vi "AddControlArray.vi"(8 "error in (no error)":errorcluster, 9 "CtlRef Array":refnum<vi>[](array[refnum]), 10 "CtlLabel Array":string[](array[string]), 11 "CtlLookup In":T1) -> (0 "error out":errorcluster, 3 "CtlLookup Out":T1)   [LabVIEW 2020, in "CtlReferences.lvlib" / "CtlReferences.lvclass"]
uses:
  CtlReferences.lvclass
  TypeDefs/CtlLookup.ctl
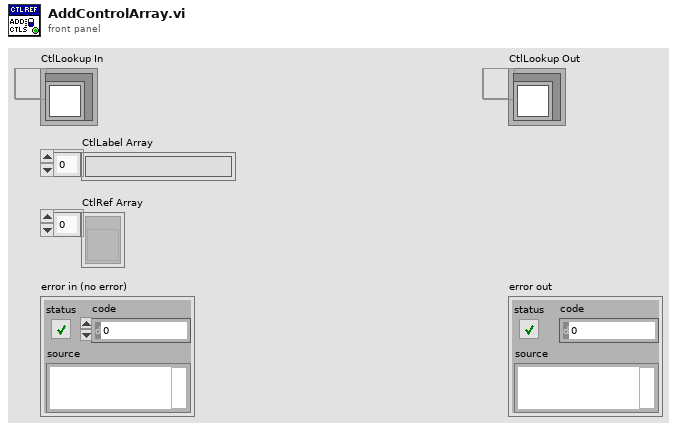
[diagram p1: front panel]
types:
  T1 = typedef "CtlReferences.lvlib/CtlReferences.lvclass/CtlLookup.ctl" = refnum<data-value>
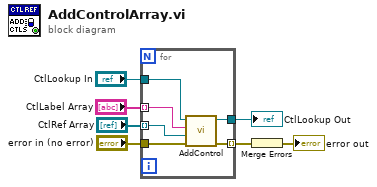
[diagram p0: block diagram]
diagram:
  n1 = for {
    tunnel: "error in (no error)" -> [w11]
    tunnel: "CtlRef Array" -> [w8] mode=indexing
    tunnel: "CtlLabel Array" -> [w9] mode=indexing
    tunnel: [w13] -> w7 mode=indexing
    tunnel: [w12] -> w3
    tunnel: "CtlLookup In" -> [w10]
    n2 = call "AddControl.vi"("error in (no error)"=w11, "CtlRef"=w8, "CtlName"=w9, "CtlLookup In"=w10) -> ("error out"=w13:errorcluster, "CtlLookup Out"=w12:T1)  [unwired: 6 in]
  }
  "CtlLookup Out" <- w3
  n3 = Merge Errors(w7) -> (→"error out":errorcluster)
